vi "json Get Structured Type Info.vi"(8 "error in (no error)":errorcluster, 10 "path":string, 11 "JSON Document in":refnum<class "JSON Document.lvclass">) -> (0 "error out":errorcluster, 1 "value out":refnum<class "JSON Document.lvclass">, 2 "count":i32, 3 "JSON Document out":refnum<class "JSON Document.lvclass">)   [LabVIEW 2015, in "JSON Document.lvclass"]
uses:
  JSON Document.lvclass
  JSON Document.lvclass/JSON Document.ctl
  rapidjson wrapper/rapidjson wrapper.lvlib
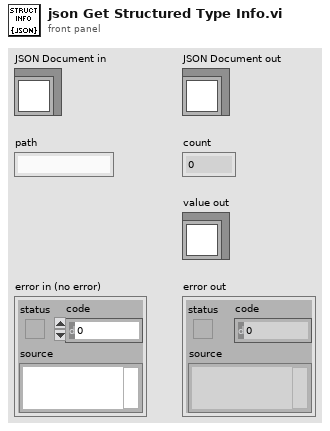
[diagram p1: front panel]
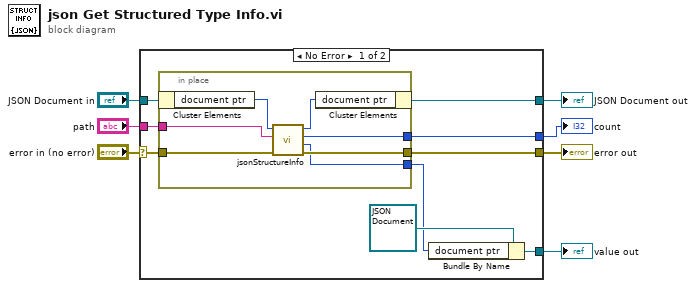
[diagram p0: block diagram]
diagram:
  n1 = case shown="No Error" "error in (no error)" {
    selector: "error in (no error)" -> [w15 w25]
    tunnel: [w14 w25] -> w6
    tunnel: [w10 w24] -> w4
    tunnel: "JSON Document in" -> [w11 w24]
    tunnel: "path" -> [w16 _]
    tunnel: [w9 _] -> w2
    tunnel: [w8 _] -> w1
    frame No Error {
      n2 = in-place {
        in-place-border: w16 -> [w21]
        in-place-border: w15 -> [w20]
        in-place-border: [w19] -> w14
        in-place-border: [w18] -> w8
        in-place-border: [w17] -> w12
        n3 = in-place-cluster #1(w11) -> ("document ptr"=w23:i64)
        n4 = call "jsonStructureInfo.vi"("error in (no error)"=w20, "path"=w21, "d in"=w23) -> ("error out"=w19:errorcluster, "value out"=w17:i64, "count"=w18:i32, "d out"=w22:i64)  [unwired: 5 in]
        n5 = in-place-cluster #1("document ptr"=w22) -> (w10:refnum<class "JSON Document.lvclass">)
      }
      n6 = Bundle By Name(cluster=refnum<class "JSON Document.lvclass"> refnum ("JSON Document in"), "document ptr"=w12) -> (w9:refnum<class "JSON Document.lvclass">)
    }
    frame Error {
    }
  }
  "error out" <- w6
  "JSON Document out" <- w4
  "count" <- w1
  "value out" <- w2
